vi "00. Native MQTT Broker.vi"() -> ()   [LabVIEW 2019]
uses:
  <vilib>/G Open Source Project for LabVIEW/MQTT Broker/PacketTracer/PacketTracer.lvclass
  <vilib>/G Open Source Project for LabVIEW/MQTT Broker/Server class/Server.lvclass/Server.ctl
  <vilib>/LabVIEW Open Source Project/MQTT Connection/MQTT_Base/Base Class/MQTT_Base.lvclass/MQTT_Base.ctl
  <vilib>/LabVIEW Open Source Project/Connection/Connection.TCP/Connection.TCP.lvclass
  C:/Program Files (x86)/National Instruments/LabVIEW 2019/vi.lib/LabVIEW Open Source Project/Connection/Connection/Connection.lvclass
  <vilib>/G Open Source Project for LabVIEW/MQTT Broker/Server class/Server.lvclass
  C:/Program Files (x86)/National Instruments/LabVIEW 2019/vi.lib/LabVIEW Open Source Project/MQTT Connection/MQTT_Base/Base Class/MQTT_Base.lvclass
  <vilib>/LabVIEW Open Source Project/MQTT Control Packets/Control Packets/PUBLISH/PUBLISH.lvclass
  C:/Program Files (x86)/National Instruments/LabVIEW 2019/vi.lib/LabVIEW Open Source Project/MQTT Control Packets/Control Packets/ControlPacket/ControlPacket.lvclass
  <vilib>/LabVIEW Open Source Project/MQTT Control Packets/Control Packets/ControlPacket/ControlPacket.lvclass
  <vilib>/LabVIEW Open Source Project/MQTT Connection/MQTT_Base/Base Class/MQTT_Base.lvclass
  <vilib>/LabVIEW Open Source Project/Connection/Connection/Connection.lvclass
panel:
  out "NbConnections":u32
  out "Inbound Message":string
  out "error server":errorcluster
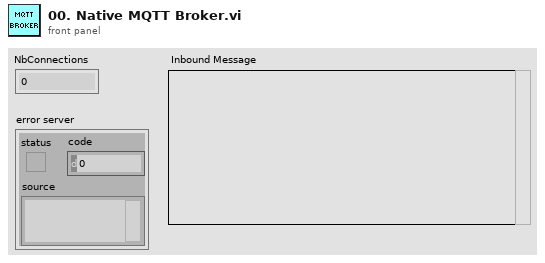
[diagram p1: front panel]
types:
  T1 = typedef "MQTT Base.lvlib/MQTT_Base.lvclass/Public Events -- cluster.ctl" = cluster{"Stop Event":refnum<user-event>, "Error Event":refnum<user-event>, "Inbound Message":refnum<user-event>}
  T2 = typedef "MQTT Server.lvlib/Server.lvclass/Public Events -- cluster.ctl" = cluster{"NbConnections":refnum<user-event>, "Client Event":refnum<user-event>}
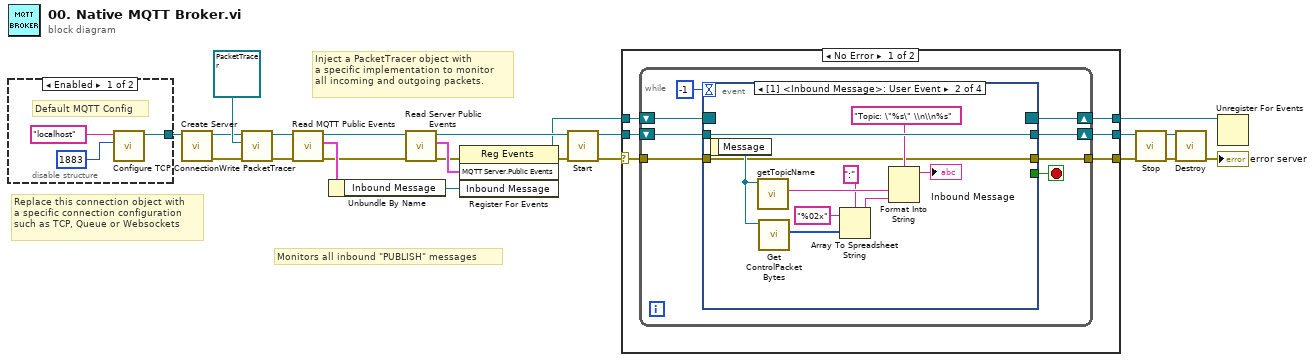
[diagram p0: block diagram]
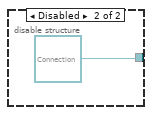
[diagram p2: hidden frame]
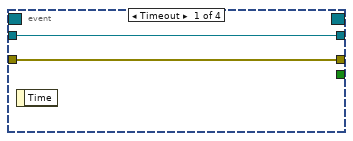
[diagram p3: hidden frame]
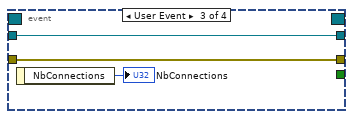
[diagram p4: hidden frame]
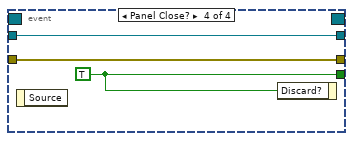
[diagram p5: hidden frame]
diagram:
  # "Replace this connection object with\na specific connection configuration\nsuch as TCP, Queue or Websockets"
  # "Inject a PacketTracer object with\na specific implementation to monitor\nall incoming and outgoing packets."
  # "Monitors all inbound \"PUBLISH\" messages"
  n1 = disable-structure shown="Enabled" {
    disable-tunnel: [w26 refnum<class "Connection.lvclass"> refnum ("Connection Configuration")] -> w23
    frame Enabled {
      # "Default MQTT Config"
      n2 = call <vilib>:"Configure TCP Connection.vi"("remote port (80)"=u16 1883, "address (localhost)"="localhost") -> ("Connection.TCP"=w26:refnum<class "Connection.TCP.lvclass">)  [unwired: 8 in, 1 out]
    }
    frame Disabled {
    }
  }
  n3 = call <vilib>:"Create Server.vi"("Connection Configuration"=w23) -> ("error out"=w20:errorcluster, "Server"=w18:refnum<class "Server.lvclass">)  [unwired: 9 in]
  n4 = call <vilib>:"Write PacketTracer.vi"("error in (no error)"=w20, "PacketTracer"=refnum<class "PacketTracer.lvclass"> refnum ("MQTT Server.lvlib:PacketTracer.lvclass"), "Server in"=w18) -> ("error out"=w21:errorcluster, "Server out"=w19:refnum<class "Server.lvclass">)  [unwired: 7 in]
  n5 = call <vilib>:"Read MQTT Public Events.vi"("error in (no error)"=w21, "MQTT_Base in"=w19) -> ("error out"=w15:errorcluster, "MQTT Public Events"=w16:T1, "MQTT_Base out"=w14:refnum<class "Server.lvclass">)  [unwired: 7 in]
  n6 = Unbundle By Name(w16) -> ("Inbound Message"=w17:refnum<user-event>)
  n7 = call <vilib>:"Read Server Public Events.vi"("error in (no error)"=w15, "Server in"=w14) -> ("error out"=w1:errorcluster, "MQTT Server.Public Events"=w2:T2, "Server out"=w5:refnum<class "Server.lvclass">)  [unwired: 7 in]
  n8 = register-events(error in=w1, w2, w17) -> (reference out=w3:refnum<event-registration>, error out=w7:errorcluster)  [unwired: 1 in]
  n9 = call <vilib>:"Start.vi"("error in (no error)"=w7, "MQTT_Base in"=w5) -> ("error out"=w8:errorcluster, "MQTT_Base out"=w6:refnum<class "Server.lvclass">)  [unwired: 7 in, 1 out]
  n10 = case shown="No Error" w8 {
    selector: w8 -> [w28 w60]
    tunnel: w6 -> [w33 w62]
    tunnel: [w32 w62] -> w11
    tunnel: w3 -> [w31 w61]
    tunnel: [w30 w61] -> w4
    tunnel: [w29 w60] -> w13
    frame No Error {
      n11 = while {
        shift-right: [w38] -> w32
        shift-left: w33 -> [w40]
        tunnel: [w35] -> w29
        tunnel: w28 -> [w34]
        shift-right: [w36] -> w30
        shift-left: w31 -> [w37]
        stop <- w39 stop-if-true
        n12 = event shown="[1] <Inbound Message>: User Event" {
          selector: w37 -> [_ _ _ _]
          dyn-events: [_ _ _ _] -> w36
          timeout: -1 -> [_ _ _ _]
          tunnel: w40 -> [w43 w53 w56 w59]
          tunnel: [_ _ _ w57] -> w39
          tunnel: [w43 w53 w56 w59] -> w38
          tunnel: [w42 w44 w54 w58] -> w35
          tunnel: w34 -> [w42 w44 w54 w58]
          event Timeout {
            n13 = event-data() -> ()  [unwired: 1 in, 1 out]
          }
          event User Event {
            n14 = event-data() -> ("Message"=w45:refnum<class "PUBLISH.lvclass">)  [unwired: 1 in]
            n15 = call <vilib>:"getTopicName.vi"("PUBLISH in"=w45) -> ("Topic"=w52:string)  [unwired: 8 in, 2 out]
            n16 = call <vilib>:"Get ControlPacket Bytes.vi"("ControlPacket"=w45) -> ("Bytes Stream"=w49:u8[])  [unwired: 7 in, 3 out]
            n17 = Array To Spreadsheet String(delimiter (Tab)=":", array=w49, 3:"%02x" ("format string")) -> (spreadsheet string=w46:string)
            n18 = Format Into String(format string="Topic: \"%s\" \\n\\n%s", w52, w46) -> (resulting string=→"Inbound Message":string)  [unwired: 2 in, 1 out]
          }
          event User Event {
            n19 = event-data() -> ("NbConnections"=→"NbConnections":u32)  [unwired: 1 in]
          }
          event Panel Close? {
            w57 = TRUE ("Discard?")
            n20 = event-data() -> ()  [unwired: 1 in, 1 out]
            n21 = event-data("Discard?"=w57) -> ()  [unwired: 1 in, 1 out]
          }
        }
      }
    }
    frame Error {
    }
  }
  n22 = call <vilib>:"Stop.vi"("error in (no error)"=w13, "MQTT_Base in"=w11) -> ("error out"=w12:errorcluster, "MQTT_Base out"=w10:refnum<class "Server.lvclass">)  [unwired: 7 in, 1 out]
  n23 = call <vilib>:"Destroy.vi"("error in (no error)"=w12, "MQTT_Base in"=w10) -> ("error out"=→"error server":errorcluster)  [unwired: 8 in, 1 out]
  n24 = Unregister For Events(event registration refnum=w4) -> ()  [unwired: 1 in, 1 out]
